vi "Send Set CANopen Master Node-ID.vi"(7 "Message Priority (Normal)":T1=enum."Normal", 8 "error in (no error)":errorcluster, 10 "Node-ID":u8=127 format="0x%02x", 11 "Message Enqueuer":refnum<class "Message Enqueuer.lvclass">) -> (0 "error out":errorcluster, 3 "Message Enqueuer out":refnum<class "Message Enqueuer.lvclass">)   [LabVIEW 2020, in "Interactor.lvlib" / "Set CANopen Master Node-ID Msg.lvclass"]
doc: "This VI sends the message to an actor."
uses:
  Set CANopen Master Node-ID Msg.lvclass
  Set CANopen Master Node-ID Msg.lvclass/Set CANopen Master Node-ID Msg.ctl
  <vilib>/ActorFramework/Message Enqueuer/Message Enqueuer.lvclass
  <vilib>/ActorFramework/Message Enqueuer/Message Priority.ctl
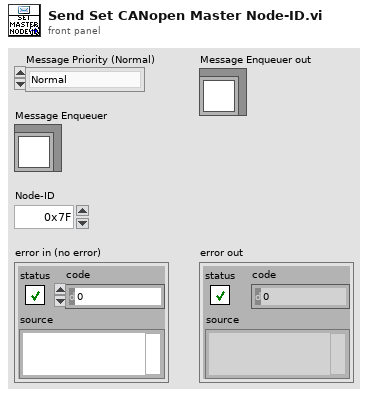
[diagram p1: front panel]
types:
  T1 = typedef "Actor Framework.lvlib/Message Enqueuer.lvclass/Message Priority.ctl" = enum16{"Low", "Normal", "High"}
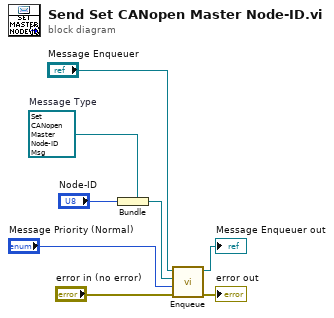
[diagram p0: block diagram]
diagram:
  w5 = refnum<class "Set CANopen Master Node-ID Msg.lvclass"> refnum  # Message Type
  n1 = Bundle(cluster=w5, "Node-ID") -> (w4:refnum<class "Set CANopen Master Node-ID Msg.lvclass">)
  n2 = call <vilib>:"Enqueue.vi"("error in (no error)"="error in (no error)", "Message Priority (Normal)"="Message Priority (Normal)", "Message"=w4, "Message Enqueuer in"="Message Enqueuer") -> ("error out"=→"error out":errorcluster, "Message Enqueuer out"=→"Message Enqueuer out":refnum<class "Message Enqueuer.lvclass">)  [unwired: 6 in]
